vi "Read Oscilloscope.lvclass.vi"(11 "Switching Time in":refnum<class "Switching Time.lvclass">) -> (2 "Oscilloscope.lvclass":refnum<class "Oscilloscope.lvclass">, 3 "Switching Time out":refnum<class "Switching Time.lvclass">)   [LabVIEW 2020, in "Switching Time.lvclass"]
uses:
  Switching Time.lvclass
  Instruments/Oscilloscope/Oscilloscope.lvclass
  Switching Time.lvclass/Switching Time.ctl
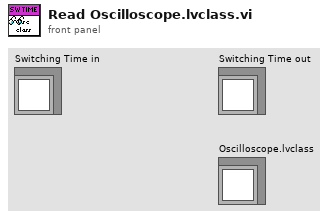
[diagram p1: front panel]
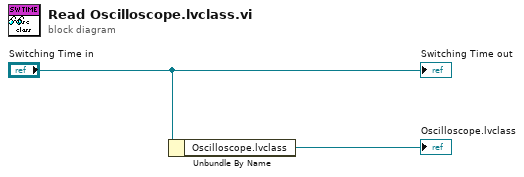
[diagram p0: block diagram]
diagram:
  n1 = Unbundle By Name("Switching Time in") -> ("Oscilloscope.lvclass"=→"Oscilloscope.lvclass":refnum<class "Oscilloscope.lvclass">)
  "Switching Time out" <- "Switching Time in"
